vi "Get Module Information.vi"(8 "error in":errorcluster, 11 "routing and faulting in":T3 format="%.0x") -> (0 "error out":errorcluster, 2 "module information":T1[](array[typedef]), 3 "routing and faulting out":T3 format="%.0x")   [LabVIEW 2020, in "Routing and Faulting Scripting.lvlib"]
uses:
  Routing and Faulting Scripting.lvlib
  <vilib>/NI VeriStand/Custom Device API/Custom Device Item Ref.ctl
  Types/Module Information.ctl
  Shared/Routing and Faulting Hardware API/Types/Possible Connections for Endpoint.ctl
  NationalInstruments.VeriStand.SystemStorage
  Shared/Routing and Faulting Hardware API/Routing and Faulting Hardware API.lvlib
  <vilib>/NI VeriStand/Custom Device API/Custom Device API.lvlib
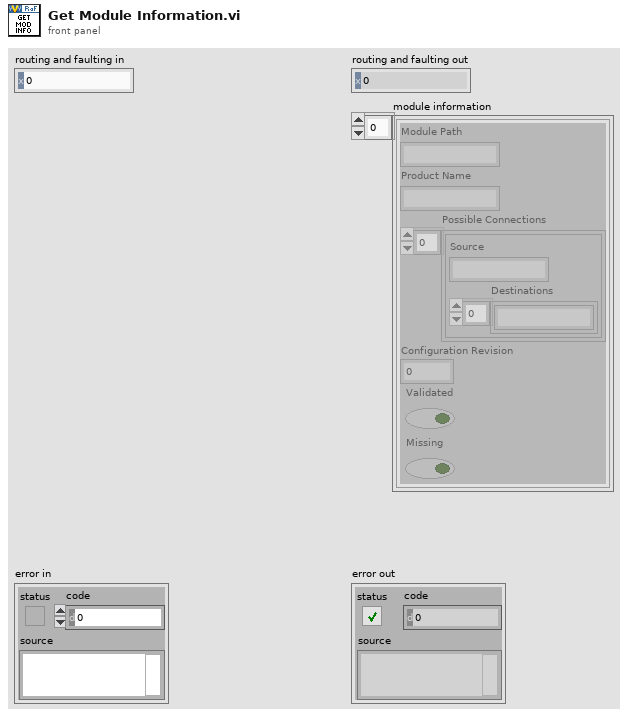
[diagram p1: front panel]
types:
  T1 = typedef "Routing and Faulting Scripting.lvlib/Module Information.ctl" = cluster{"Module Path":string, "Product Name":string, "Possible Connections":T2[], "Configuration Revision":u32, "Validated":bool, "Missing":bool}
  T2 = typedef "Routing and Faulting Hardware API.lvlib/Possible Connections for Endpoint.ctl" = cluster{"Source":string, "Destinations":string[]}
  T3 = typedef "Custom Device API.lvlib/Custom Device Item Ref.ctl" = u64
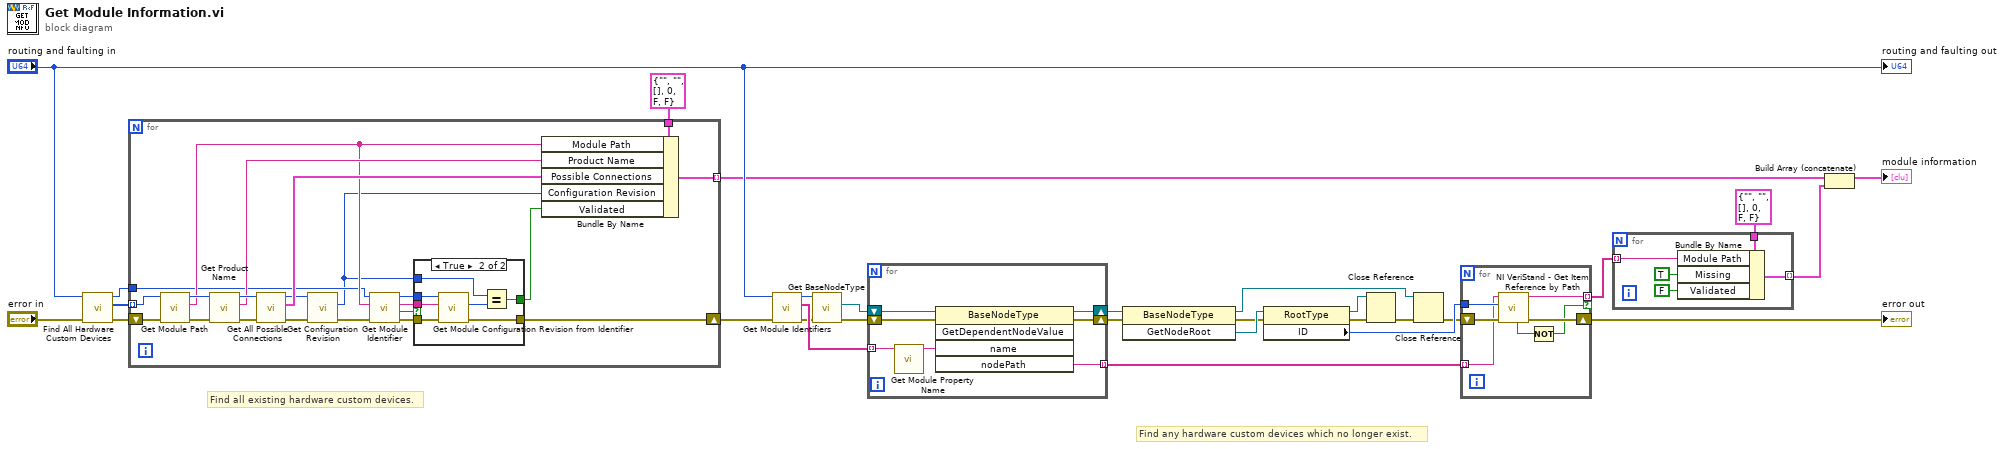
[diagram p0: block diagram]
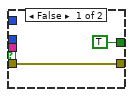
[diagram p2: hidden frame]
diagram:
  # "Find any hardware custom devices which no longer exist."
  # "Find all existing hardware custom devices."
  n1 = call "Find All Hardware Custom Devices.vi"("error in (no error)"="error in", "Routing and Faulting Ref in"="routing and faulting in") -> ("error out"=w28:errorcluster, "Hardware Refs"=w27:T3[], "Routing and Faulting Ref out"=w25:T3)  [unwired: 7 in]
  n2 = for {
    shift-right: [w32] -> w19
    shift-left: w28 -> [w51]
    tunnel: w27 -> [w48] mode=indexing
    tunnel: T1 {"Module Path"="", "Product Name"="", "Possible Connections"=[], "Configuration Revision"=0, "Validated"=FALSE, "Missing"=FALSE} ("Module Connection Information") -> [w47]
    tunnel: [w42] -> w16 mode=indexing
    tunnel: w25 -> [w37]
    n3 = call "Get Module Path.vi"("error in (no error)"=w51, "Hardware Ref in"=w48) -> ("error out"=w50:errorcluster, "Module Path"=w38:string, "Hardware Ref out"=w46:T3)  [unwired: 6 in, 1 out]
    n4 = call "Get Product Name.vi"("error in (no error)"=w50, "Hardware Ref in"=w46) -> ("error out"=w49:errorcluster, "Product Name"=w44:string, "Hardware Ref out"=w45:T3)  [unwired: 6 in, 1 out]
    n5 = call "Get All Possible Connections.vi"("error in (no error)"=w49, "Hardware Ref in"=w45) -> ("error out"=w41:errorcluster, "Possible Connections"=w43:T2[], "Hardware Ref out"=w40:T3)  [unwired: 6 in, 1 out]
    n6 = call "Get Configuration Revision.vi"("error in (no error)"=w41, "Hardware Ref in"=w40) -> ("error out"=w39:errorcluster, "Configuration Revision"=w30:u32)  [unwired: 6 in, 2 out]
    n7 = call "Get Module Identifier.vi"("error in"=w39, "module path"=w38, "routing and faulting in"=w37) -> ("error out"=w35:errorcluster, "found?"=w31:bool, "module identifier"=w34:string, "routing and faulting out"=w33:T3)  [unwired: 5 in]
    n8 = case shown="True" w31 {
      tunnel: [TRUE w60] -> w36
      tunnel: w35 -> [w52 w59]
      tunnel: w34 -> [_ w58]
      tunnel: w33 -> [_ w57]
      tunnel: [w52 w55] -> w32
      tunnel: w30 -> [_ w54]
      frame False {
      }
      frame True {
        n9 = call "Get Module Configuration Revision from Identifier.vi"("error in"=w59, "module identifier"=w58, "routing and faulting in"=w57) -> ("error out"=w55:errorcluster, "configuration revision"=w56:u32)  [unwired: 6 in, 1 out]
        n10 = Equal?(x=w54, y=w56) -> (x = y?=w60:bool)
      }
    }
    n11 = Bundle By Name(cluster=w47, "Module Path"=w38, "Product Name"=w44, "Possible Connections"=w43, "Configuration Revision"=w30, "Validated"=w36) -> (w42:T1)
  }
  n12 = call "Get Module Identifiers.vi"("error in"=w19, "routing and faulting in"="routing and faulting in") -> ("error out"=w22:errorcluster, "module Identifier"=w24:string[], "routing and faulting out"=w20:T3)  [unwired: 7 in]
  n13 = call "Get BaseNodeType.vi"("error in"=w22, "item in"=w20) -> ("error out"=w21:errorcluster, "BaseNodeType"=w23:refnum<k24>)  [unwired: 7 in, 1 out]
  n14 = for {
    tunnel: w24 -> [w62] mode=indexing
    shift-right: [w65] -> w10
    shift-left: w21 -> [w67]
    shift-right: [w64] -> w9
    shift-left: w23 -> [w66]
    tunnel: [w61] -> w18 mode=indexing
    n15 = call "Get Module Property Name.vi"("module identifier"=w62) -> ("module property name"=w63:string)  [unwired: 10 in]
    n16 = invoke class="BaseNodeType" method="GetDependentNodeValue"(reference=w66, error in=w67, "name"=w63) -> (reference out=w64:refnum<k24>, error out=w65:errorcluster, "nodePath"=w61:string)  [unwired: 2 in, 2 out]
  }
  n17 = invoke class="BaseNodeType" method="GetNodeRoot"(reference=w9, error in=w10) -> (reference out=w8:refnum<k24>, error out=w6:errorcluster, "GetNodeRoot"=w7:refnum<k24>)  [unwired: 1 in]
  n18 = property class="RootType"(reference=w7, error in=w6) -> (reference out=w3:refnum<k24>, error out=w4:errorcluster, "ID"=w2:u64)
  n19 = Close Reference(reference=w3, error in (no error)=w4) -> (error out=w5:errorcluster)
  n20 = Close Reference(reference=w8, error in (no error)=w5) -> (error out=w1:errorcluster)
  n21 = for {
    tunnel: w2 -> [w73]
    shift-right: [w72] -> w14
    shift-left: w1 -> [w74]
    tunnel: w18 -> [w71] mode=indexing
    tunnel: [w70] -> w13 mode=indexing if=w68
    n22 = call <vilib>:"NI VeriStand - Get Item Reference by Path.vi"("error in (no error)"=w74, "Root Ref"=w73, "Item Path in"=w71) -> ("error out"=w72:errorcluster, "Item Path out"=w70:string, "Found"=w69:bool)  [unwired: 5 in, 1 out]
    n23 = Not(x=w69) -> (.not. x?=w68:bool)
  }
  "error out" <- w14
  n24 = for {
    tunnel: w13 -> [w78] mode=indexing
    tunnel: T1 {"Module Path"="", "Product Name"="", "Possible Connections"=[], "Configuration Revision"=0, "Validated"=FALSE, "Missing"=FALSE} ("Module Connection Information") -> [w79]
    tunnel: [w76] -> w11 mode=indexing
    n25 = Bundle By Name(cluster=w79, "Module Path"=w78, "Missing"=TRUE ("Validated"), "Validated"=FALSE) -> (w76:T1)
  }
  n26 = Build Array (concatenate)(w16, w11) -> (→"module information":T1[])
  "routing and faulting out" <- "routing and faulting in"
